vi "INI Signer.vi"(1 "String Key Values":string) -> (0 "Signature":string)   [LabVIEW 2017]
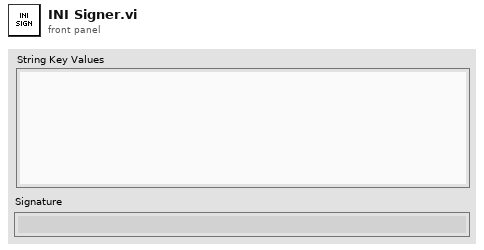
[diagram p1: front panel]
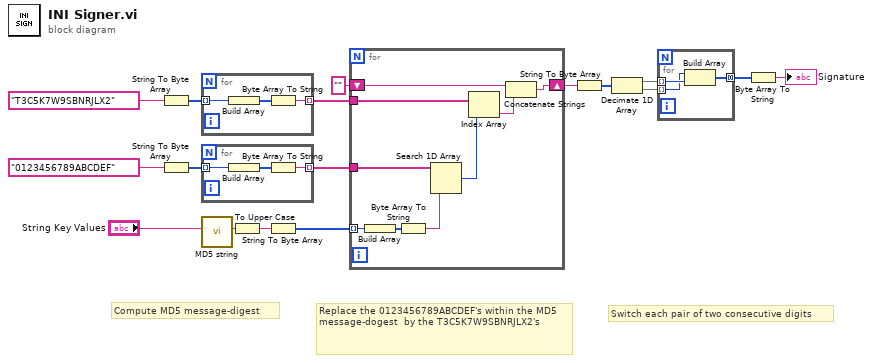
[diagram p0: block diagram]
diagram:
  # "Switch each pair of two consecutive digits"
  # "Compute MD5 message-digest"
  # "Replace the 0123456789ABCDEF's within the MD5 message-dogest  by the T3C5K7W9SBNRJLX2's"
  n1 = String To Byte Array(string="T3C5K7W9SBNRJLX2" ("Message String")) -> (unsigned byte array=w15:u8[])
  n2 = String To Byte Array(string="0123456789ABCDEF" ("Message String")) -> (unsigned byte array=w12:u8[])
  n3 = for {
    tunnel: w15 -> [w20] mode=indexing
    tunnel: [w18] -> w10 mode=indexing
    n4 = Build Array(w20) -> (w19:u8[])
    n5 = Byte Array To String(unsigned byte array=w19) -> (string=w18:string)
  }
  n6 = for {
    tunnel: w12 -> [w23] mode=indexing
    tunnel: [w21] -> w11 mode=indexing
    n7 = Build Array(w23) -> (w22:u8[])
    n8 = Byte Array To String(unsigned byte array=w22) -> (string=w21:string)
  }
  n9 = call "MD5 string.vi"("Message String"="String Key Values") -> ("MD5 message-digest"=w17:string)  [unwired: 10 in]
  n10 = To Upper Case(1:w17) -> (0:w8:string)
  n11 = String To Byte Array(string=w8) -> (unsigned byte array=w16:u8[])
  n12 = for {
    tunnel: w16 -> [w32] mode=indexing
    tunnel: w11 -> [w30]
    tunnel: w10 -> [w29]
    shift-right: [w27] -> w7
    shift-left: "" -> [w26]
    n13 = Build Array(w32) -> (w31:u8[])
    n14 = Byte Array To String(unsigned byte array=w31) -> (string=w24:string)
    n15 = Search 1D Array(1D array=w30, element=w24) -> (index of element=w25:i32)  [unwired: 1 in]
    n16 = Index Array(array=w29, index=w25) -> (element=w28:string)
    n17 = Concatenate Strings(w26, w28) -> (w27:string)
  }
  n18 = String To Byte Array(string=w7) -> (unsigned byte array=w2:u8[])
  n19 = Decimate 1D Array(w2) -> (w6:u8[], w5:u8[])
  n20 = for {
    tunnel: w6 -> [w35] mode=indexing
    tunnel: w5 -> [w34] mode=indexing
    tunnel: [w33] -> w4 mode=concatenating
    n21 = Build Array(w34, w35) -> (w33:u8[])
  }
  n22 = Byte Array To String(unsigned byte array=w4) -> (string=→"Signature":string)
